vi "Checkers P1 King Drawer.vi"() -> (3 "new picture":picture)   [LabVIEW 2014]
uses:
  Game Info Global Variable.vi
types:
  T1 = cluster{"Font Name:":string, "Size":i16, "Strikeout?":bool, "Italic?":bool, "Underline?":bool, "Outline?":bool, "Shadow?":bool, "Bold?":bool}
  T2 = cluster{"left":i16, "top":i16, "right":i16, "bottom":i16}
  T3 = enum16{"User-specified Font", "Application Font", "System Font", "Dialog Font"}
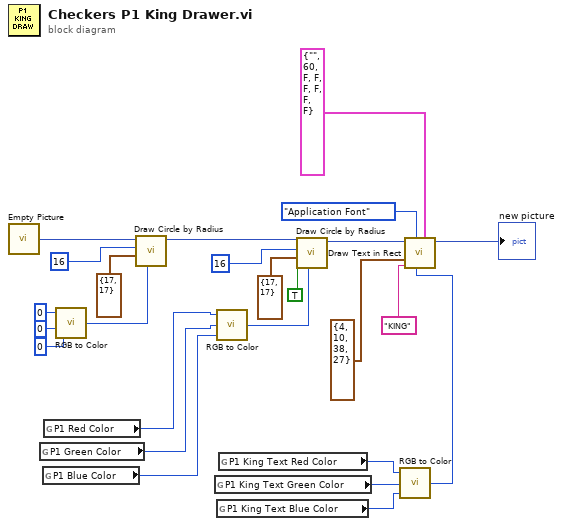
[diagram p0: block diagram]
diagram:
  n1 = call "Empty Picture"() -> ("empty picture"=w22:picture)
  n2 = global read "Game Info Global Variable.vi" "P1 Green Color"() -> (w6:i32)
  n3 = global read "Game Info Global Variable.vi" "P1 Blue Color"() -> (w7:i32)
  n4 = global read "Game Info Global Variable.vi" "P1 Red Color"() -> (w5:i32)
  n5 = call <vilib>:"RGB to Color.vi"("B"=u8 0, "G"=u8 0, "R"=u8 0) -> ("Color"=w25:u32)
  n6 = call <vilib>:"Draw Circle by Radius.vi"("color(black)"=w25, "pixel center"=cluster{"horizontal":i16, "vertical":i16} {"horizontal"=17, "vertical"=17}, "radius"=i16 16, "picture"=w22) -> ("new picture"=w15:picture)  [unwired: 7 in]
  n7 = global read "Game Info Global Variable.vi" "P1 King Text Green Color"() -> (w2:i32)
  n8 = call <vilib>:"RGB to Color.vi"("B"=w7, "G"=w6, "R"=w5) -> ("Color"=w16:u32)
  n9 = global read "Game Info Global Variable.vi" "P1 King Text Blue Color"() -> (w1:i32)
  n10 = global read "Game Info Global Variable.vi" "P1 King Text Red Color"() -> (w3:i32)
  n11 = call <vilib>:"Draw Circle by Radius.vi"("color(black)"=w16, "fill?(F)"=TRUE, "pixel center"=cluster{"horizontal":i16, "vertical":i16} {"horizontal"=17, "vertical"=17}, "radius"=i16 16, "picture"=w15) -> ("new picture"=w13:picture)  [unwired: 6 in]
  n12 = call <vilib>:"RGB to Color.vi"("B"=w1, "G"=w2, "R"=w3) -> ("Color"=w4:u32)
  n13 = call <vilib>:"Draw Text in Rect.vi"("[user-specified font]"=T1 {"Font Name:"="", "Size"=60, "Strikeout?"=FALSE, "Italic?"=FALSE, "Underline?"=FALSE, "Outline?"=FALSE, "Shadow?"=FALSE, "Bold?"=FALSE}, "text color(black)"=w4, "desired font(Application)"=T3."Application Font", "text"="KING", "rect"=T2 {"left"=4, "top"=10, "right"=38, "bottom"=27}, "picture"=w13) -> ("new picture"=→"new picture":picture)  [unwired: 5 in]
